vi "niRFUtil MT UTIL Apply Frequency Offset (Internal).vi"   [LabVIEW 2015, in "niRFUtil.lvlib"]
uses:
  niRFUtil.lvlib
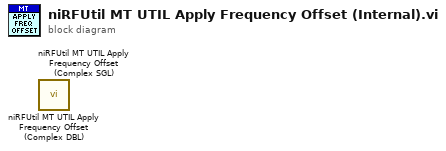
[diagram p0: block diagram]
diagram:
  n1 = call "niRFUtil MT UTIL Apply Frequency Offset (Complex DBL).vi"() -> ()  [unwired: 14 in, 2 out]
  n2 = call "niRFUtil MT UTIL Apply Frequency Offset (Complex SGL).vi"() -> ()  [unwired: 14 in, 2 out]
